vi "Array-Make Strings Unique.vi"(3 "Use parentheses":bool, 4 "Strings":string[](array[string])) -> (1 "Unique Strings":string[](array[string]))   [LabVIEW 2020]
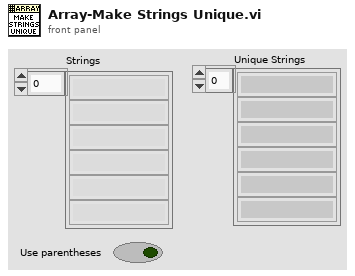
[diagram p1: front panel]
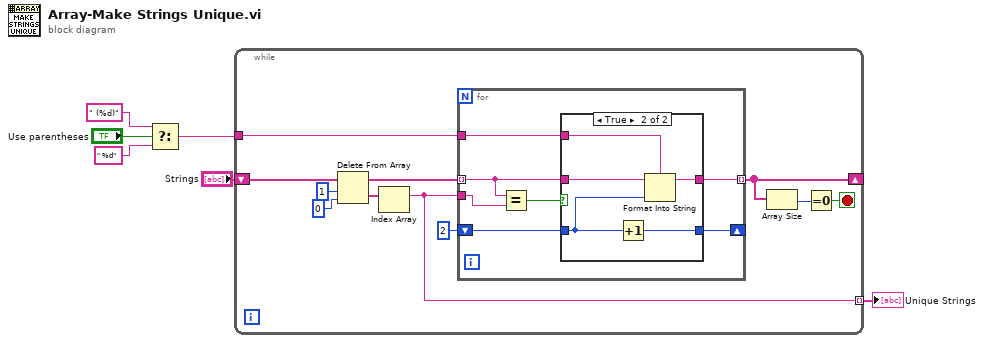
[diagram p0: block diagram]
diagram:
  n1 = Select(t=" (%d)" ("format string"), s="Use parentheses", f=" %d" ("format string")) -> (s? t:f=w2:string)
  n2 = while {
    shift-right: [w13] -> _
    shift-left: "Strings" -> [w17]
    tunnel: [w12] -> w5 mode=indexing
    tunnel: w2 -> [w7]
    stop <- w11 stop-if-true
    n3 = Delete From Array(array=w17, length=1, index=0) -> (deleted portion=w15:string[], array with subset deleted=w14:string[])
    n4 = Index Array(array=w15) -> (element=w12:string)  [unwired: 1 in]
    n5 = for {
      tunnel: w12 -> [w24]
      tunnel: w14 -> [w22] mode=indexing
      tunnel: [w21] -> w13 mode=indexing
      shift-right: [w19] -> _
      shift-left: 2 -> [w20]
      tunnel: w7 -> [w18]
      n6 = Equal?(x=w22, y=w24) -> (x = y?=w23:bool)
      n7 = case shown="True" w23 {
        tunnel: w22 -> [w26 w31]
        tunnel: [w26 w30] -> w21
        tunnel: w20 -> [w25 w29]
        tunnel: [w25 w28] -> w19
        tunnel: w18 -> [_ w27]
        frame False {
        }
        frame True {
          n8 = Increment(x=w29) -> (x+1=w28:i32)
          n9 = Format Into String(format string=w27, initial string=w31, w29) -> (resulting string=w30:string)  [unwired: 1 in, 1 out]
        }
      }
    }
    n10 = Array Size(array=w13) -> (size(s)=w10:i32)
    n11 = Equal To 0?(x=w10) -> (x = 0?=w11:bool)
  }
  "Unique Strings" <- w5
